vi "Recieve Request for Result.vi"(6 "Request time":timestamp, 8 "error in (no error)":errorcluster, 9 "Requestor":string, 10 "Requestee":string, 11 "Mag Lab Measure Controller in":refnum<class "Mag Lab Measure Controller.lvclass">) -> (0 "error out":errorcluster, 3 "Mag Lab Measure Controller out":refnum<class "Mag Lab Measure Controller.lvclass">)   [LabVIEW 2015, in "Mag Lab Measure Controller.lvclass"]
uses:
  Mag Lab Measure Controller.lvclass
  Mag Lab Root/Mag Lab Root.lvclass/Mag Lab Root.ctl
  Mag Lab Root Messages/Recieve Request for Result Msg/Recieve Request for Result Msg.lvclass/Recieve Request for Result Msg.ctl
  <vilib>/ActorFramework/Message Enqueuer/Message Enqueuer.lvclass/Message Enqueuer.ctl
  <vilib>/ActorFramework/Message Enqueuer/Enqueue.vi
  <vilib>/ActorFramework/Message Priority Queue/Priority Enqueue.vi
  Mag Lab Root Messages/Recieve Request for Result Msg/Recieve Request for Result Msg.lvclass
  Compound Measurement/Compound Measurement.lvclass
  Mag Lab Measure Base/Mag Lab Measure Base.lvclass
  Mag Lab Root/Mag Lab Root.lvclass
  Mag Lab Error Handler/Mag Lab Error Handler.lvclass
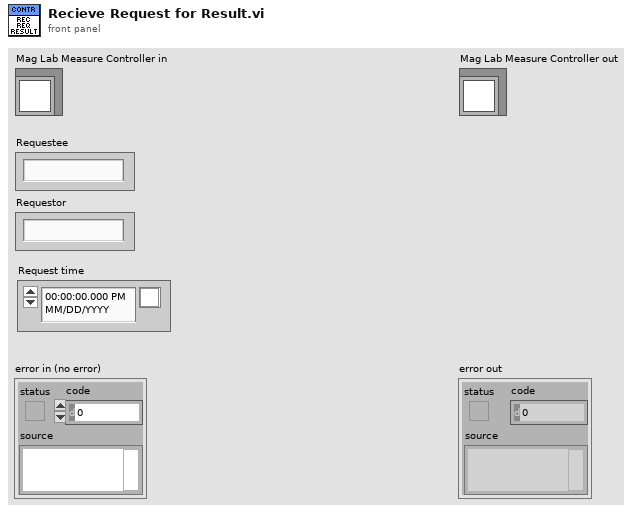
[diagram p1: front panel]
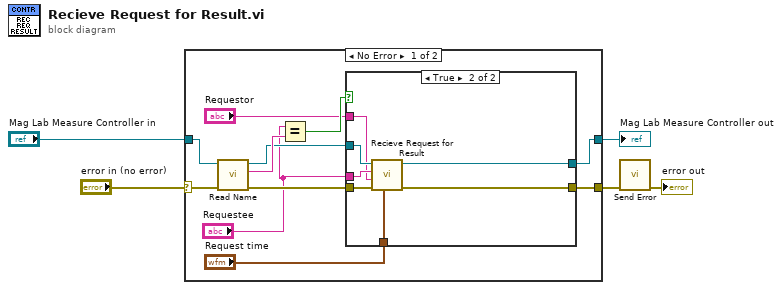
[diagram p0: block diagram]
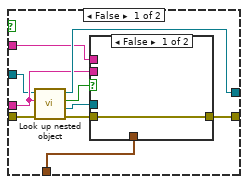
[diagram p2: hidden frame]
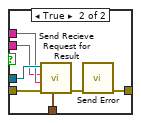
[diagram p3: hidden frame]
diagram:
  n1 = case shown="No Error" "error in (no error)" {
    selector: "error in (no error)" -> [w12 w43]
    tunnel: [w16 w43] -> w2
    tunnel: [w15 w42] -> w3
    tunnel: "Mag Lab Measure Controller in" -> [w14 w42]
    frame No Error {
      n2 = call "Read Name.vi"("error in (no error)"=w12, "Mag Lab Root in"=w14) -> ("error out"=w11:errorcluster, "Name"=w13:string, "Mag Lab Root out"=w9:refnum<class "Mag Lab Measure Controller.lvclass">)  [unwired: 7 in]
      n3 = Equal?(x="Requestee", y=w13) -> (x = y?=w10:bool)
      n4 = case shown="True" w10 {
        tunnel: [w24 w37] -> w16
        tunnel: [w23 w36] -> w15
        tunnel: "Requestor" -> [w22 w38]
        tunnel: "Requestee" -> [w20 w39]
        tunnel: w11 -> [w19 w41]
        tunnel: w9 -> [w18 w40]
        tunnel: "Request time" -> [w17 w35]
        frame False {
          n5 = call "Look up nested object.vi"("error in (no error)"=w19, "Object name"=w20, "Mag Lab Measure Base in"=w18) -> ("error out"=w25:errorcluster, "Object Queue"=w26:refnum<class "Message Enqueuer.lvclass">, "Found?"=w21:bool, "Mag Lab Measure Base out"=w23:refnum<class "Mag Lab Measure Controller.lvclass">)  [unwired: 5 in]
          n6 = case shown="False" w21 {
            tunnel: w26 -> [_ w34]
            tunnel: w25 -> [w27 w33]
            tunnel: [w27 w29] -> w24
            tunnel: w22 -> [_ w32]
            tunnel: w20 -> [_ w31]
            tunnel: w17 -> [_ w28]
            frame False {
            }
            frame True {
              n7 = call "Send Recieve Request for Result.vi"("Request time"=w28, "error in (no error)"=w33, "Requestor"=w32, "Requestee"=w31, "Message Enqueuer"=w34) -> ("error out"=w30:errorcluster)  [unwired: 5 in, 1 out]
              n8 = call "Send Error.vi"("error in (no error)"=w30) -> ("error out"=w29:errorcluster)  [unwired: 9 in, 1 out]
            }
          }
        }
        frame True {
          n9 = call-parent "Recieve Request for Result.vi"("Request time"=w35, "error in (no error)"=w41, "Requestor"=w38, "Requestee"=w39, "Compound Measurement in"=w40) -> ("error out"=w37:errorcluster, "Compound Measurement out"=w36:refnum<class "Mag Lab Measure Controller.lvclass">)  [unwired: 5 in]
        }
      }
    }
    frame Error {
    }
  }
  "Mag Lab Measure Controller out" <- w3
  n10 = call "Send Error.vi"("error in (no error)"=w2) -> ("error out"=→"error out":errorcluster)  [unwired: 9 in, 1 out]
